vi "SENS_PATH_CONF_CAT.vi"(0 "VISA IN":refnum<visa-resource-name>, 5 "error in":errorcluster) -> (13 "Data":string[](array[string]), 14 "VISA Out":refnum<visa-resource-name>, 16 "Response":string, 19 "error out":errorcluster)   [LabVIEW 2018, in "PNA-X.lvlib"]
doc: "SENSe:PATH:CONFiguration:DELete <string>\n(Write-only) Deletes the specified configuration name from the PNA. The factory configurations cannot be deleted. This is the only method of distinguishing a factory configuration from a user-named configuration.\n \nParameters\n \n \n<string>\n Configuration name to be deleted.\n \nExamples\n SENS:PATH:CONF:DEL \"MyMixer\"\n \nReturn Type\n Not Applicable\n \nDefault\n Not Applicable"
uses:
  PNA-X.lvlib
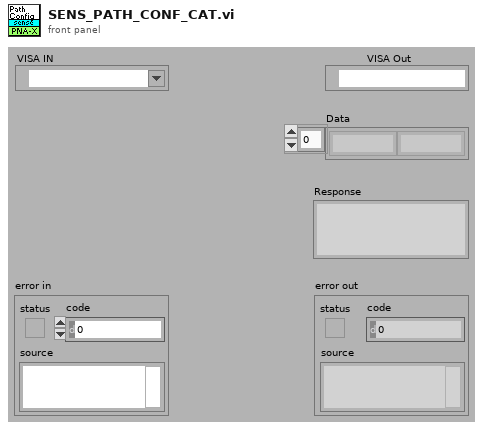
[diagram p1: front panel]
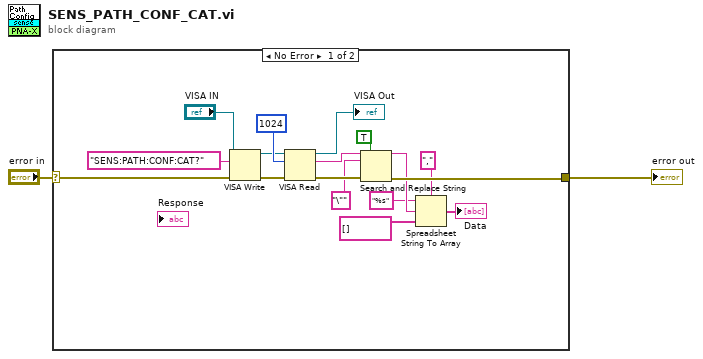
[diagram p0: block diagram]
diagram:
  n1 = case shown="No Error" "error in" {
    selector: "error in" -> [w14 w20]
    tunnel: [w11 w20] -> w1
    frame No Error {
      n2 = VISA Write(VISA resource name="VISA IN", write buffer="SENS:PATH:CONF:CAT?" ("Cmdline"), error in (no error)=w14) -> (VISA resource name out=w16:refnum<visa-resource-name>, error out=w18:errorcluster)  [unwired: 1 out]
      n3 = VISA Read(VISA resource name=w16, byte count=1024, error in (no error)=w18) -> (VISA resource name out=→"VISA Out":refnum<visa-resource-name>, read buffer=w10:string, error out=w12:errorcluster)  [unwired: 1 out]
      n4 = Search and Replace String(replace all?=TRUE ("replace all? (F)"), input string=w10, search string="\"", error in=w12) -> (result string=w7:string, error out=w11:errorcluster)  [unwired: 4 in, 2 out]
      n5 = Spreadsheet String To Array(delimiter (Tab)=",", format string="%s", spreadsheet string=w7, array type (2D Dbl)=string[] []) -> (array=→"Data":string[])
    }
    frame Error {
    }
  }
  "error out" <- w1
